vi "MarginBottom.vi"(1 "输入":u32[][](array[numeric])) -> (0 "输出":i32)   [LabVIEW 2010]
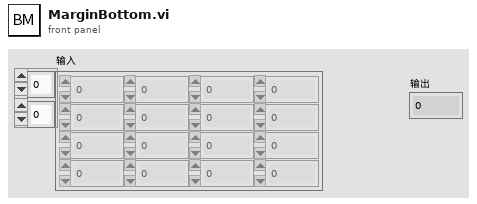
[diagram p1: front panel]
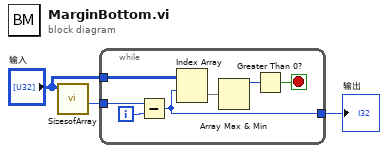
[diagram p0: block diagram]
diagram:
  n1 = call "SizesofArray.vi"("数组"="输入") -> ("NumRows_r"=w1:i32)  [unwired: 7 in, 3 out]
  n2 = while {
    tunnel: "输入" -> [w10]
    tunnel: [w7] -> w3
    tunnel: w1 -> [w4]
    i -> [w8]
    stop <- w5 stop-if-true
    n3 = Subtract(x=w4, y=w8) -> (x-y=w7:i32)
    n4 = Index Array(array=w10, index (row)=w7) -> (element=w9:u32[])  [unwired: 1 in]
    n5 = Array Max & Min(array=w9) -> (max value=w6:u32)  [unwired: 3 out]
    n6 = Greater Than 0?(x=w6) -> (x > 0?=w5:bool)
  }
  "输出" <- w3
